vi "Get Sender.vi"(11 "Setup Msg in":refnum<class "Setup Msg.lvclass">) -> (2 "Sender":refnum<class "Sender.lvclass">)   [LabVIEW 2021, in "jettl.lvlib" / "Setup Msg.lvlib" / "Setup Msg.lvclass"]
uses:
  Setup Msg.lvclass
  Sender/Sender/Sender.lvclass
  Setup Msg.lvclass/Setup Msg.ctl
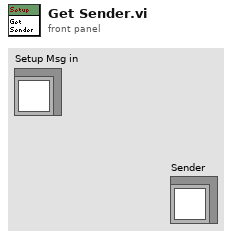
[diagram p1: front panel]
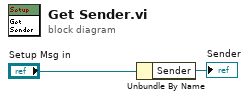
[diagram p0: block diagram]
diagram:
  n1 = Unbundle By Name("Setup Msg in") -> ("Sender"=→"Sender":refnum<class "Sender.lvclass">)
